vi "EvaluateSecondsTrigger.vi"(7 "trigger":i32, 10 "seconds":i32) -> (2 "output":bool)   [LabVIEW 2017, in "CronScheduler.lvlib"]
uses:
  <vilib>/addons/InsightCM/Utilities/CronScheduler/CronScheduler.lvlib
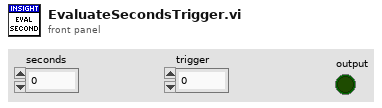
[diagram p1: front panel]
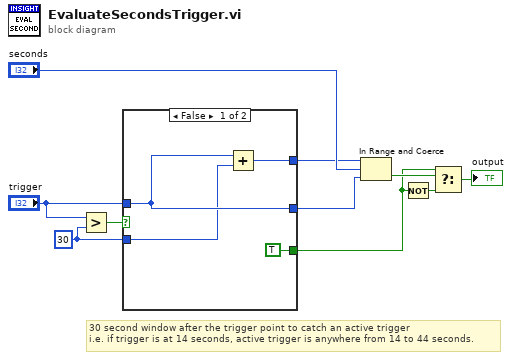
[diagram p0: block diagram]
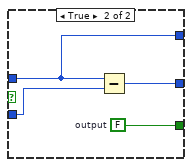
[diagram p2: hidden frame]
diagram:
  w1 = 30 ("y")
  # "30 second window after the trigger point to catch an active trigger\ni.e. if trigger is at 14 seconds, active trigger is anywhere from 14 to 44 seconds."
  n1 = Greater?(x="trigger", y=w1) -> (0:w10:bool)
  n2 = case shown="False" w10 {
    tunnel: "trigger" -> [w12 w15]
    tunnel: [w13 w15] -> w7
    tunnel: [w12 w18] -> w6
    tunnel: [TRUE ("output") w17] -> w3
    tunnel: w1 -> [w11 w16]
    frame False {
      n3 = Add(x=w12, y=w11) -> (x+y=w13:i32)
    }
    frame True {
      w17 = FALSE  # output
      n4 = Subtract(x=w15, y=w16) -> (x-y=w18:i32)
    }
  }
  n5 = In Range and Coerce(upper limit=w7, x="seconds", lower limit=w6) -> (In Range?=w5:bool)  [unwired: 1 out]
  n6 = Not(x=w3) -> (.not. x?=w4:bool)
  n7 = Select(t=w3, s=w5, f=w4) -> (s? t:f=→"output":bool)
